vi "PCAN_VERSION.vi"(8 "error in (no error)":errorcluster) -> (0 "error out":errorcluster, 2 "lpszTextBuff":string, 3 "error":T1 items=["CAN_ERR_OK"=0, "CAN_ERR_XMTFULL"=1, "CAN_ERR_OVERRUN"=2, "CAN_ERR_BUSLIGHT"=4, "CAN_ERR_BUSHEAVY"=8, "CAN_ERR_BUSOFF"=16, "CAN_ERR_QRCVEMPTY"=32, "CAN_ERR_QOVERRUN"=64, "CAN_ERR_QXMTFULL"=128, "CAN_ERR_REGTEST"=256, "CAN_ERR_NOVXD"=512, "CAN_ERR_RESOURCE"=8192, "CAN_ERR_ILLPARAMTYPE"=16384, "CAN_ERR_ILLPARAMVAL"=32768])   [LabVIEW 2016]
uses:
  PCAN_ERROR.ctl
  PCAN_USB.DLL
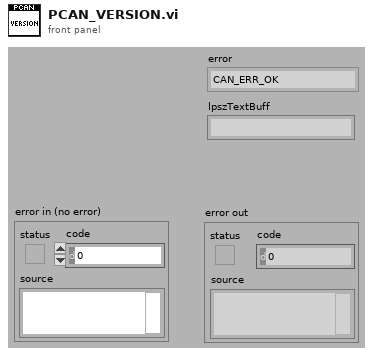
[diagram p1: front panel]
types:
  T1 = typedef "PCAN_ERROR.ctl" = i32
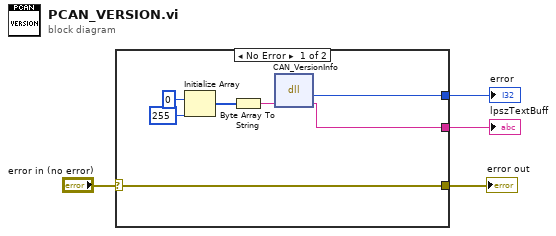
[diagram p0: block diagram]
diagram:
  n1 = case shown="No Error" "error in (no error)" {
    selector: "error in (no error)" -> [w10 w12]
    tunnel: [w11 _] -> w2
    tunnel: [w10 w12] -> w3
    tunnel: [w5 _] -> w1
    frame No Error {
      n2 = Initialize Array(u8 0 ("element"), 255 ("dimension size")) -> (w7:u8[])
      n3 = Byte Array To String(unsigned byte array=w7) -> (string=w6:string)
      n4 = dll-call lib="D:/LabView/08_PCAN&Measurement/PCAN_Driver/PCAN_USB.DLL" fn="CAN_VersionInfo"("lpszTextBuff"=w6) -> ("return type"=w11:i32, "lpszTextBuff"=w5:string)  [unwired: 3 in, 2 out]
    }
    frame Error {
    }
  }
  "error out" <- w3
  "error" <- w2
  "lpszTextBuff" <- w1
